vi "Variant to Attribute.vi"(8 "error in (no error)":errorcluster, 10 "Parameter":variant, 11 "Number Msg in":refnum<class "Number Msg.lvclass">) -> (0 "error out":errorcluster, 3 "Number Msg out":refnum<class "Number Msg.lvclass">)   [LabVIEW 2015, in "TestLNA.lvlib" / "Number Msg.lvclass"]
doc: "Read message attributes from parameter variant.\n\n<b>Attention:</b> This dynamic dispatch VI was added to the Message.lvclass in order to provide a mechnism to allow for generic parameter parsing. Refer to CS++LNA.lvlib:CS++LNAMessage.lvclass.Do.vi"
uses:
  Number Msg.lvclass
  Number Msg.lvclass/Number Msg.ctl
  <vilib>/ActorFramework/Message/Message.lvclass
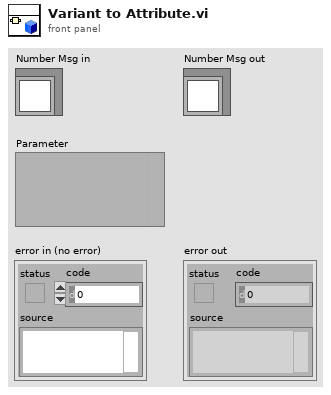
[diagram p1: front panel]
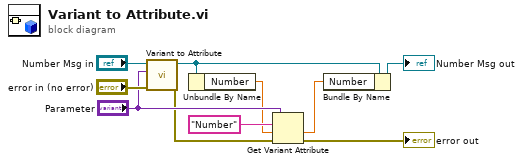
[diagram p0: block diagram]
diagram:
  n1 = call-parent "Variant to Attribute.vi"("error in (no error)"="error in (no error)", "Parameter"="Parameter", "Message in"="Number Msg in") -> ("error out"=w6:errorcluster, "Message out"=w3:refnum<class "Number Msg.lvclass">)  [unwired: 7 in]
  n2 = Unbundle By Name(w3) -> ("Number"=w4:dbl)
  n3 = Get Variant Attribute(Variant="Parameter", name="Number", default value (empty Variant)=w4, error in=w6) -> (value=w1:dbl, error out=→"error out":errorcluster)  [unwired: 2 out]
  n4 = Bundle By Name(cluster=w3, "Number"=w1) -> (→"Number Msg out":refnum<class "Number Msg.lvclass">)
